vi "Setup UI.vi"(8 "error in (no error)":errorcluster, 10 "Set UI to input? (F)":bool, 11 "Magnetic Field Lakeshore Continuous in":refnum<class "Magnetic Field Lakeshore Continuous.lvclass">) -> (0 "error out":errorcluster, 3 "Magnetic Field Lakeshore Continuous out":refnum<class "Magnetic Field Lakeshore Continuous.lvclass">)   [LabVIEW 2017, in "Magnetic Field Lakeshore Continuous.lvclass"]
doc: "Scanner::Setup is a constructor that has no parameters and faces the user. The Factory calls this VI to let the user configure this Scanner. It is dynamically dispatched in order to let the user choose the type as well as the options of the scanner."
uses:
  Magnetic Field Lakeshore Continuous.lvclass
  Magnetic Field Lakeshore Continuous.lvclass/Magnetic Field Lakeshore Continuous.ctl
  Instruments/Utility Classes/Scannable/Scannable.lvclass
panel:
  in  "Go to first field":bool
  in  "Go to setpoint set":bool
  in  "Setpoint Set":dbl[unit]
  out "Current Setpoint":dbl[unit]
  in  "Field control on/off toggle":bool
  in  "Control slope limit":dbl[unit]=0.16666666666666666
  in  "Integral":dbl[unit]=1.0
  in  "Proportional":dbl=10.0
  in  "Field reading":dbl[unit]
  in  "Set control parameters":bool
  out "Suggested dwell time per point":dbl[unit]
  in  "specifyrate":bool=TRUE
  in  "Total Time for Scan":dbl[unit]
  in  "Ramp rate":dbl[unit]
  # "Continuous B Field Scan\n(Lakeshore Gaussmeter)"
  # "Note: the scan parameters above must be in Gauss"
  # "This needs to be on before you do the scan or select \"Go to first point\"!"
  # "specify by sweep rate"
  # "specify by total time"
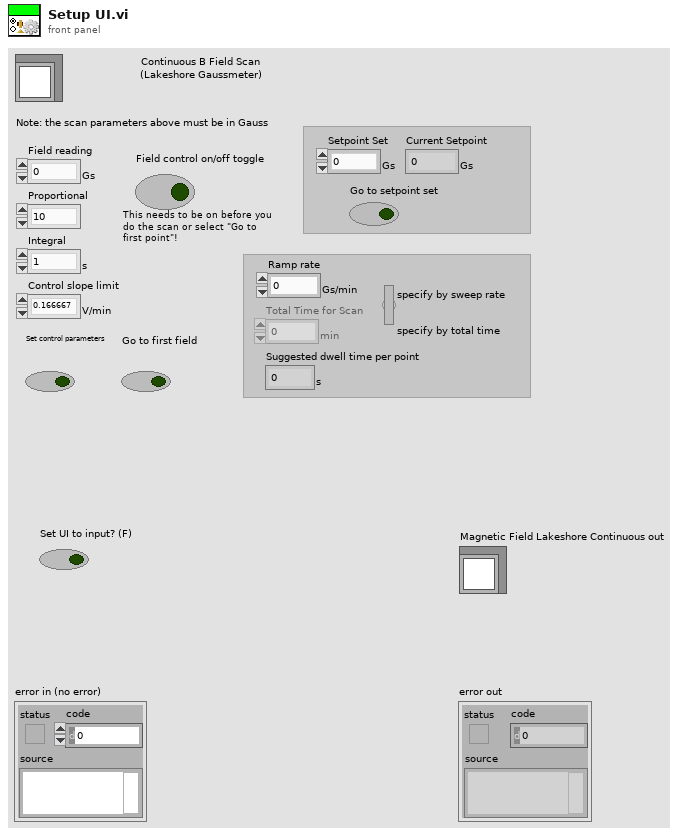
[diagram p1: front panel]
types:
  T1 = typedef "Scanner.lvclass/Range.ctl" = cluster{"xi":dbl, "xf":dbl, "dx":dbl, "Return to...?":bool, "Return to":dbl}
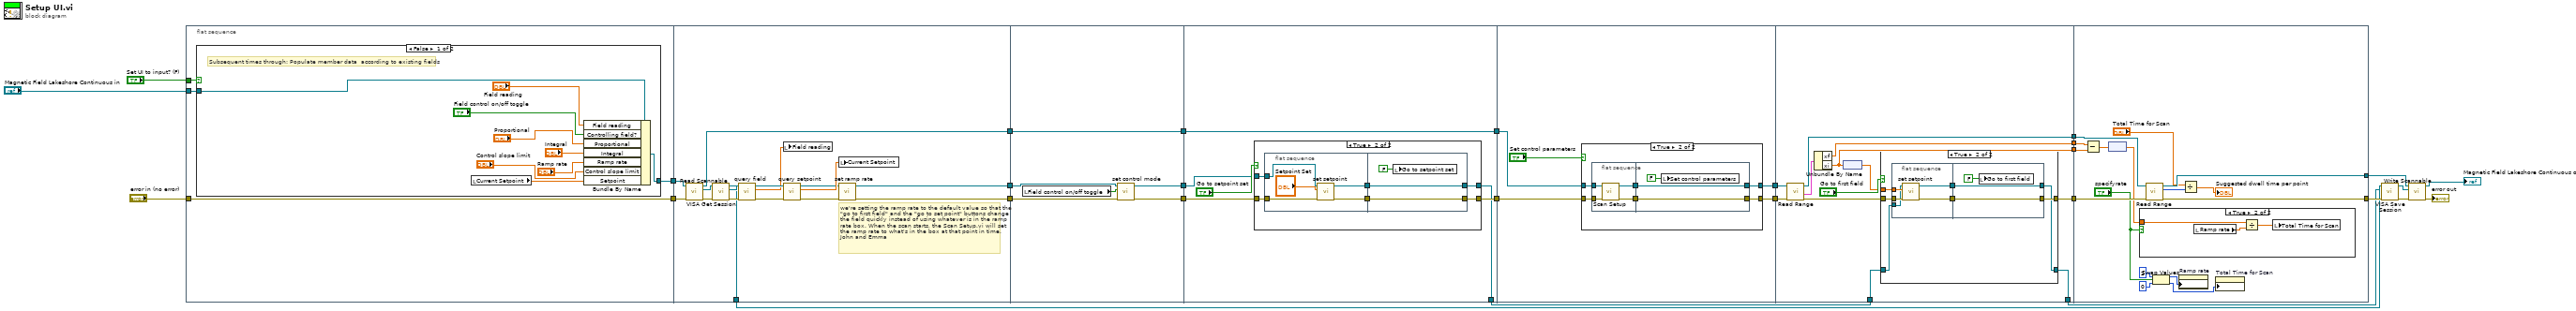
[diagram p0: block diagram]
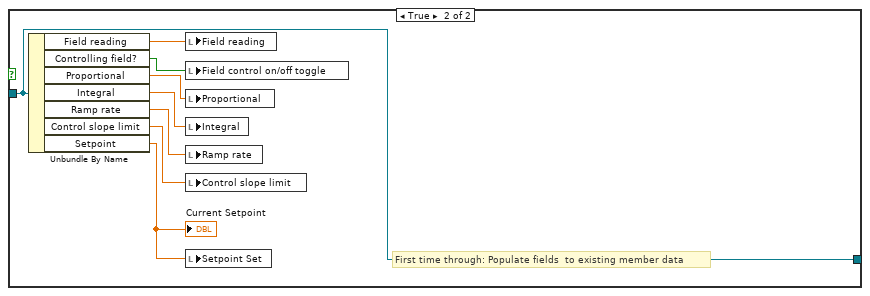
[diagram p2: hidden frame]
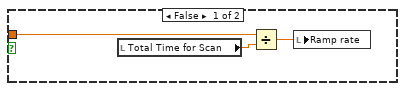
[diagram p6: hidden frame]
diagram:
  n1 = flat-sequence {
    tunnel: [w32] -> w25
    tunnel: "error in (no error)" -> [w32]
    tunnel: [w31] -> w24
    tunnel: "Magnetic Field Lakeshore Continuous in" -> [w30]
    tunnel: "Set UI to input? (F)" -> [w29]
    tunnel: w25 -> [w59]
    tunnel: [w50] -> w23
    tunnel: w24 -> [w58]
    tunnel: [w57] -> w22
    tunnel: [w52] -> w21
    tunnel: [w54] -> w12
    tunnel: w23 -> [w69]
    tunnel: [w68] -> w20
    tunnel: w22 -> [w71]
    tunnel: [w71] -> w19
    tunnel: w21 -> [w70]
    tunnel: [w66] -> w18
    tunnel: w20 -> [w74]
    tunnel: [w73] -> w17
    tunnel: w19 -> [w77]
    tunnel: [w77] -> w16
    tunnel: w18 -> [w75]
    tunnel: [w72] -> w5
    tunnel: w17 -> [w95]
    tunnel: [w94] -> w8
    tunnel: w16 -> [w97]
    tunnel: [w96] -> w7
    tunnel: w8 -> [w123]
    tunnel: w7 -> [w122]
    tunnel: [w121] -> w6
    tunnel: w5 -> [w124]
    tunnel: [w114] -> w4
    tunnel: [w118] -> w3
    tunnel: [w116] -> w2
    tunnel: [w115] -> w1
    tunnel: w6 -> [w158]
    tunnel: [w146] -> w13
    tunnel: [w156] -> w11
    tunnel: w3 -> [w157]
    tunnel: w2 -> [w144]
    tunnel: w1 -> [w143]
    frame #0 {
      n2 = case shown="False" w29 {
        tunnel: [w40 w49] -> w31
        tunnel: w30 -> [w41 w49]
        frame False {
          # "Subsequent times through: Populate member data  according to existing fields"
          n3 = local read "Current Setpoint"() -> (w33:dbl[unit])
          n4 = Bundle By Name(cluster=w41, "Field reading"="Field reading", "Controlling field?"="Field control on/off toggle", "Proportional"="Proportional", "Integral"="Integral", "Ramp rate"="Ramp rate", "Control slope limit"="Control slope limit", "Setpoint"=w33) -> (w40:refnum<class "Magnetic Field Lakeshore Continuous.lvclass">)
        }
        frame True {
          # "First time through: Populate fields  to existing member data"
          n5 = Unbundle By Name(w49) -> ("Field reading"=w47:dbl[unit], "Controlling field?"=w46:bool, "Proportional"=w45:dbl, "Integral"=w44:dbl[unit], "Ramp rate"=w48:dbl[unit], "Control slope limit"=w43:dbl[unit], "Setpoint"=w42:dbl[unit])
          "Current Setpoint" <- w42
          n6 = local write "Field reading"(w47) -> ()
          n7 = local write "Field control on/off toggle"(w46) -> ()
          n8 = local write "Proportional"(w45) -> ()
          n9 = local write "Integral"(w44) -> ()
          n10 = local write "Ramp rate"(w48) -> ()
          n11 = local write "Control slope limit"(w43) -> ()
          n12 = local write "Setpoint Set"(w42) -> ()
        }
      }
    }
    frame #1 {
      # "we're setting the ramp rate to the default value so that the \"go to first field\" and the \"go to set point\" buttons change the field quickly instead of using whatever is in the ramp rate box. When the scan starts, the Scan Setup.vi will set the ramp rate to what's in the box at that point in time.  John and Emma"
      n13 = call-dynamic "Read Scannable.vi"("error in (no error)"=w59, "Scanner.lvclass in"=w58) -> ("error out"=w65:errorcluster, "Scannable.lvclass"=w64:refnum<class "Scannable.lvclass">, "Scanner.lvclass out"=w57:refnum<class "Magnetic Field Lakeshore Continuous.lvclass">)  [unwired: 7 out]
      n14 = call-dynamic "VISA Get Session.vi"("error in (no error)"=w65, "Instrument.lvclass in"=w64) -> ("error out"=w62:errorcluster, "VISA Resource Name"=w63:refnum<visa-resource-name>, "Instrument.lvclass out"=w54:refnum<class "Scannable.lvclass">)  [unwired: 7 out]
      n15 = call "query field.vi"("error in (no error)"=w62, "VISA session"=w63) -> ("error out"=w60:errorcluster, "Field reading"=w56:dbl[unit], "dup VISA session"=w61:refnum<visa-resource-name>)  [unwired: 7 in]
      n16 = local write "Field reading"(w56) -> ()
      n17 = call "query setpoint.vi"("error in (no error)"=w60, "VISA session"=w61) -> ("error out"=w51:errorcluster, "Setpoint"=w55:dbl[unit], "dup VISA session"=w53:refnum<visa-resource-name>)  [unwired: 7 in]
      n18 = local write "Current Setpoint"(w55) -> ()
      n19 = call "set ramp rate.vi"("error in (no error)"=w51, "VISA session"=w53) -> ("error out"=w50:errorcluster, "dup VISA session"=w52:refnum<visa-resource-name>)  [unwired: 8 in]
    }
    frame #2 {
      n20 = local read "Field control on/off toggle"() -> (w67:bool)
      n21 = call "set control mode.vi"("error in (no error)"=w69, "Start/stop controlling field"=w67, "VISA session"=w70) -> ("error out"=w68:errorcluster, "dup VISA session"=w66:refnum<visa-resource-name>)  [unwired: 7 in]
    }
    frame #3 {
      n22 = case shown="True" "Go to setpoint set" {
        tunnel: w75 -> [w79 w85]
        tunnel: w74 -> [w78 w84]
        tunnel: [w78 w83] -> w73
        tunnel: [w79 w82] -> w72
        frame False {
        }
        frame True {
          n23 = flat-sequence {
            tunnel: w85 -> [w89]
            tunnel: w84 -> [w87]
            tunnel: [w88] -> w81
            tunnel: [w86] -> w80
            tunnel: [w93] -> w83
            tunnel: [w91] -> w82
            tunnel: w81 -> [w91]
            tunnel: w80 -> [w93]
            frame #0 {
              n24 = call "set setpoint.vi"("error in (no error)"=w87, "Setpoint"="Setpoint Set", "VISA session"=w89) -> ("error out"=w86:errorcluster, "dup VISA session"=w88:refnum<visa-resource-name>)  [unwired: 7 in]
            }
            frame #1 {
              n25 = local write "Go to setpoint set"(FALSE ("Go to setpoint set")) -> ()
            }
          }
        }
      }
    }
    frame #4 {
      n26 = case shown="True" "Set control parameters" {
        tunnel: w97 -> [w100 w106]
        tunnel: [w100 w105] -> w96
        tunnel: w95 -> [w99 w103]
        tunnel: [w99 w102] -> w94
        frame False {
        }
        frame True {
          n27 = flat-sequence {
            tunnel: w106 -> [w110]
            tunnel: [w108] -> w104
            tunnel: w103 -> [w109]
            tunnel: [w107] -> w101
            tunnel: [w112] -> w105
            tunnel: w104 -> [w112]
            tunnel: [w111] -> w102
            tunnel: w101 -> [w111]
            frame #0 {
              n28 = call-dynamic "Scan Setup.vi"("error in (no error)"=w109, "Magnetic Field Lakeshore Continuous in"=w110) -> ("error out"=w107:errorcluster, "Magnetic Field Lakeshore Continuous out"=w108:refnum<class "Magnetic Field Lakeshore Continuous.lvclass">)  [unwired: 8 in]
            }
            frame #1 {
              n29 = local write "Set control parameters"(FALSE ("Go to first point (can't see it change!)")) -> ()
            }
          }
        }
      }
    }
    frame #5 {
      n30 = call-dynamic "Read Range.vi"("error in (no error)"=w123, "Scanner.lvclass in"=w122) -> ("error out"=w119:errorcluster, "Range"=w117:T1, "Scanner.lvclass out"=w121:refnum<class "Magnetic Field Lakeshore Continuous.lvclass">)  [unwired: 7 out]
      n31 = Unbundle By Name(w117) -> ("xf"=w116:dbl, "xi"=w115:dbl)
      n32 = node(w115) -> (w120:dbl[unit])
      n33 = case shown="True" "Go to first field" {
        tunnel: [w127 w134] -> w118
        tunnel: w124 -> [w126 w132]
        tunnel: w120 -> [_ w131]
        tunnel: w119 -> [w127 w130]
        tunnel: [w126 w129] -> w114
        frame False {
        }
        frame True {
          n34 = flat-sequence {
            tunnel: [w137] -> w133
            tunnel: w132 -> [w136]
            tunnel: w131 -> [w139]
            tunnel: w130 -> [w138]
            tunnel: [w135] -> w128
            tunnel: [w141] -> w134
            tunnel: w133 -> [w141]
            tunnel: [w140] -> w129
            tunnel: w128 -> [w140]
            frame #0 {
              n35 = call "set setpoint.vi"("error in (no error)"=w138, "Setpoint"=w139, "VISA session"=w136) -> ("error out"=w137:errorcluster, "dup VISA session"=w135:refnum<visa-resource-name>)  [unwired: 7 in]
            }
            frame #1 {
              n36 = local write "Go to first field"(FALSE ("Go to first point (can't see it change!)")) -> ()
            }
          }
        }
      }
    }
    frame #6 {
      n37 = Subtract(x=w144, y=w143) -> (x-y=w155:dbl)
      n38 = node(w155) -> (w154:dbl[unit])
      n39 = case shown="True" "specifyrate" {
        tunnel: w154 -> [w160 w163]
        frame False {
          n40 = local read "Total Time for Scan"() -> (w161:dbl[unit])
          n41 = Divide(x=w160, y=w161) -> (x/y=w159:dbl[unit])
          n42 = local write "Ramp rate"(w159) -> ()
        }
        frame True {
          n43 = local read "Ramp rate"() -> (w164:dbl[unit])
          n44 = Divide(x=w163, y=w164) -> (x/y=w162:dbl[unit])
          n45 = local write "Total Time for Scan"(w162) -> ()
        }
      }
      n46 = call-dynamic "Read Range.vi"("error in (no error)"=w157, "Scanner.lvclass in"=w158) -> ("error out"=w146:errorcluster, "# Points"=w147:u32, "Scanner.lvclass out"=w156:refnum<class "Magnetic Field Lakeshore Continuous.lvclass">)  [unwired: 7 out]
      n47 = Swap Values(12:2 ("y"), 13:"specifyrate", 14:0 ("x")) -> (1:w151:i32, 3:w150:i32)
      n48 = property on="Ramp rate" class="DigNum (strict)"("DisabledEnum"=w151) -> ()  [unwired: 2 in, 2 out]
      n49 = Divide(x="Total Time for Scan", y=w147) -> (x/y=→"Suggested dwell time per point":dbl[unit])
      n50 = property on="Total Time for Scan" class="DigNum (strict)"("DisabledEnum"=w150) -> ()  [unwired: 2 in, 2 out]
    }
  }
  n51 = call-dynamic "VISA Save Session.vi"("error in (no error)"=w13, "VISA Resource Name"=w4, "Instrument.lvclass in"=w12) -> ("error out"=w15:errorcluster, "Instrument.lvclass out"=w9:refnum<class "Scannable.lvclass">)  [unwired: 7 out]
  n52 = call-dynamic "Write Scannable.vi"("error in (no error)"=w15, "Scannable.lvclass"=w9, "Scanner.lvclass in"=w11) -> ("error out"=→"error out":errorcluster, "Scanner.lvclass out"=→"Magnetic Field Lakeshore Continuous out":refnum<class "Magnetic Field Lakeshore Continuous.lvclass">)  [unwired: 7 out]
